vi "StageSettings.vi"(1 "Get/Set":bool, 2 "PI Stage Setup (input)":T1={"channels (x, y, z)"="2,3,4", "Stage Scaling (V/µm)"=0.1} {"Stage Scaling (V/µm)" format="%.2f"}) -> (0 "PI Stage Setup (output)":T1={"channels (x, y, z)"="2,3,4", "Stage Scaling (V/µm)"=0.1} {"Stage Scaling (V/µm)" format="%.2f"})   [LabVIEW 2009]
uses:
  StageSettings.ctt
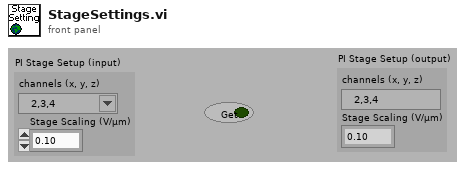
[diagram p1: front panel]
types:
  T1 = typedef "StageSettings.ctt" = cluster{"channels (x, y, z)":tag, "Stage Scaling (V/µm)":dbl}
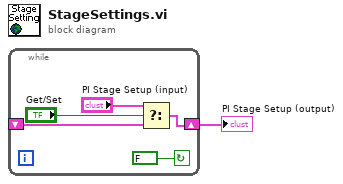
[diagram p0: block diagram]
diagram:
  n1 = while {
    shift-right: [w2] -> w1
    shift-left: _ -> [w3]
    stop <- FALSE continue-if-true
    n2 = Select(t="PI Stage Setup (input)", s="Get/Set", f=w3) -> (s? t:f=w2:T1)
  }
  "PI Stage Setup (output)" <- w1
